vi "序号加一子vi.vi"() -> (3 "当日序号":string)   [LabVIEW 2014]
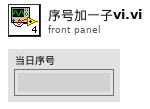
[diagram p1: front panel]
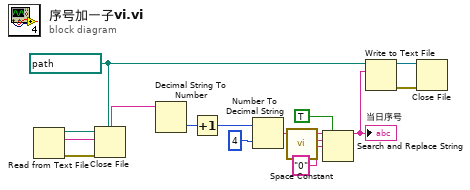
[diagram p0: block diagram]
diagram:
  w14 = path "D:/序号.txt" ("文件（使用对话框）")
  n1 = Read from Text File(file (use dialog)=w14) -> (refnum out=w4:refnum<file>, text=w5:string, error out=w3:errorcluster)  [unwired: 3 in, 1 out]
  n2 = Close File(refnum=w4, error in=w3) -> ()  [unwired: 2 out]
  n3 = Decimal String To Number(string=w5) -> (number=w11:i32)  [unwired: 2 in, 1 out]
  n4 = Increment(x=w11) -> (x+1=w12:i32)
  n5 = Number To Decimal String(number=w12, width (-)=i16 4 ("宽度(-)")) -> (decimal integer string=w7:string)
  n6 = call <vilib>:"Space Constant.vi"() -> ("String"=w10:string)
  n7 = Search and Replace String(replace all?=TRUE ("替换全部？(F)"), input string=w7, search string=w10, replace string="0" ("替换字符串(\"\")")) -> (result string=w13:string)  [unwired: 4 in, 3 out]
  "当日序号" <- w13
  n8 = Write to Text File(file (use dialog)=w14, text=w13) -> (refnum out=w1:refnum<file>, error out=w2:errorcluster)  [unwired: 2 in, 1 out]
  n9 = Close File(refnum=w1, error in=w2) -> ()  [unwired: 2 out]
